vi "Three way slider -CAT.vi"() -> ()   [LabVIEW 2012]
uses:
  CAT.ctl
panel:
  out "Mode":cluster{"Run":bool, "Hold":bool, "Off":bool}={"Run"=FALSE, "Hold"=FALSE, "Off"=TRUE}
  in  "Cluster":T1 max=2 scale=0.0..2.0
  in  "stop":bool
  out "HOLD":bool
  out "OFF":bool
  out "RUN":bool
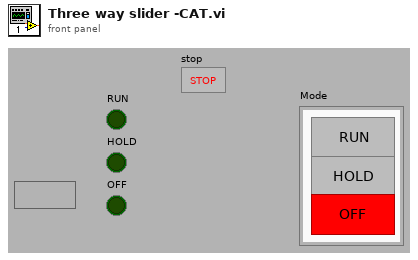
[diagram p1: front panel]
types:
  T1 = typedef "CAT.ctl" = u8
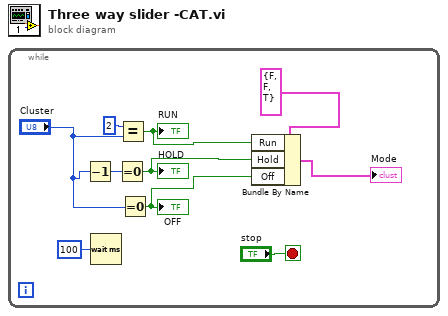
[diagram p0: block diagram]
diagram:
  n1 = while {
    stop <- "stop" stop-if-true
    n2 = Decrement(x="Cluster") -> (x-1=w8:T1)
    n3 = Wait (ms)(milliseconds to wait=u32 100) -> ()  [unwired: 1 out]
    n4 = Equal To 0?(x=w8) -> (x = 0?=w3:bool)
    "HOLD" <- w3
    n5 = Equal?(x=u32 2, y="Cluster") -> (x = y?=w2:bool)
    "RUN" <- w2
    n6 = Equal To 0?(x="Cluster") -> (x = 0?=w4:bool)
    "OFF" <- w4
    n7 = Bundle By Name(cluster=cluster{"Run":bool, "Hold":bool, "Off":bool} {"Run"=FALSE, "Hold"=FALSE, "Off"=TRUE} ("Mode"), "Run"=w2, "Hold"=w3, "Off"=w4) -> (→"Mode":cluster{"Run":bool, "Hold":bool, "Off":bool})
  }
